vi "Map 1st Generation.vi"(8 "error in":errorcluster, 11 "XML Document in":refnum<class "XML Document.lvclass">) -> (0 "error out":errorcluster, 3 "XML Document out":refnum<class "XML Document.lvclass">)   [LabVIEW 2014, in "XML Document.lvclass"]
uses:
  XML Document.lvclass
  Node_class/Node.lvclass
  <vilib>/xml/Close Reference(Node).vi
  <resource>/objmgr/DOMUserDefRef.rc
  Element_class/Element.lvclass
  <vilib>/xml/NI_XML.lvlib
  Text Node_class/Text Node.lvclass
  Comment Node_class/Comment Node.lvclass
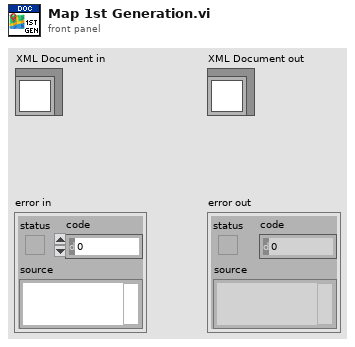
[diagram p1: front panel]
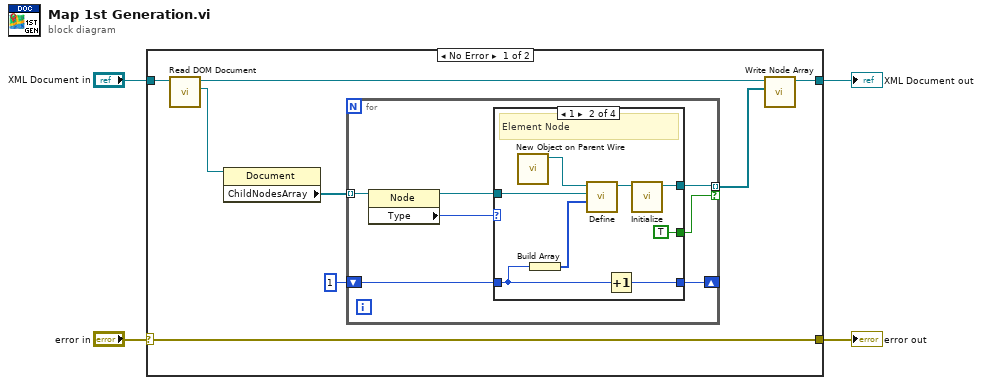
[diagram p0: block diagram]
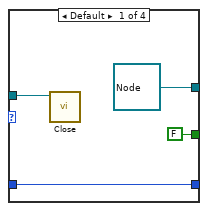
[diagram p2: hidden frame]
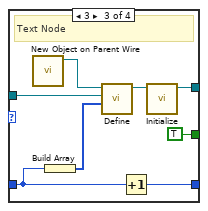
[diagram p3: hidden frame]
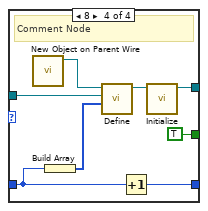
[diagram p4: hidden frame]
diagram:
  n1 = case shown="No Error" "error in" {
    selector: "error in" -> [w11 w49]
    tunnel: [w11 w49] -> w3
    tunnel: [w6 w48] -> w1
    tunnel: "XML Document in" -> [w12 w48]
    frame No Error {
      n2 = call-dynamic "Read DOM Document.vi"("XML Document in"=w12) -> ("DOM Document"=w9:refnum<k20>, "XML Document out"=w10:refnum<class "XML Document.lvclass">)  [unwired: 8 in, 1 out]
      n3 = property class="Document"(reference=w9) -> ("ChildNodesArray"=w8:refnum<k20>[])  [unwired: 1 in, 2 out]
      n4 = for {
        tunnel: w8 -> [w19] mode=indexing
        shift-right: [w15] -> _
        shift-left: 1 ("Address Location Part") -> [w16]
        tunnel: [w14] -> w5 mode=indexing if=w13
        n5 = property class="Node"(reference=w19) -> (reference out=w18:refnum<k20>, "Type"=w17:i32)  [unwired: 1 in, 1 out]
        n6 = case shown="1" w17 {
          tunnel: w18 -> [w20 w29 w37 w45]
          tunnel: w16 -> [w23 w31 w39 w47]
          tunnel: [w23 w30 w38 w46] -> w15
          tunnel: [refnum<class "Node.lvclass"> refnum ("Node out") w24 w33 w41] -> w14
          tunnel: [FALSE TRUE TRUE TRUE] -> w13
          frame Default {
            n7 = call-poly <vilib>:"Close.vi"("node"=w20) -> ()  [unwired: 8 in, 1 out]
          }
          frame 1 {
            # "Element Node"
            n8 = call "New Object on Parent Wire.vi"() -> ("Node.lvclass"=w27:refnum<class "Node.lvclass">)  [unwired: 10 in, 1 out]
            n9 = Build Array(w31) -> (w28:i32[])
            n10 = call-dynamic "Define.vi"("Address"=w28, "Node Refnum"=w29, "Node in"=w27) -> ("Node out"=w26:refnum<class "Node.lvclass">)  [unwired: 7 in, 1 out]
            n11 = Increment(x=w31) -> (x+1=w30:i32)
            n12 = call-dynamic "Initialize.vi"("Node in"=w26) -> ("Node out"=w24:refnum<class "Node.lvclass">)  [unwired: 9 in, 1 out]
          }
          frame 3 {
            # "Text Node"
            n13 = call "New Object on Parent Wire.vi"() -> ("Node.lvclass"=w35:refnum<class "Node.lvclass">)  [unwired: 10 in, 1 out]
            n14 = Build Array(w39) -> (w36:i32[])
            n15 = call-dynamic "Define.vi"("Address"=w36, "Node Refnum"=w37, "Node in"=w35) -> ("Node out"=w34:refnum<class "Node.lvclass">)  [unwired: 7 in, 1 out]
            n16 = Increment(x=w39) -> (x+1=w38:i32)
            n17 = call-dynamic "Initialize.vi"("Node in"=w34) -> ("Node out"=w33:refnum<class "Node.lvclass">)  [unwired: 9 in, 1 out]
          }
          frame 8 {
            # "Comment Node"
            n18 = call "New Object on Parent Wire.vi"() -> ("Node.lvclass"=w43:refnum<class "Node.lvclass">)  [unwired: 10 in, 1 out]
            n19 = Build Array(w47) -> (w44:i32[])
            n20 = call-dynamic "Define.vi"("Address"=w44, "Node Refnum"=w45, "Node in"=w43) -> ("Node out"=w42:refnum<class "Node.lvclass">)  [unwired: 7 in, 1 out]
            n21 = Increment(x=w47) -> (x+1=w46:i32)
            n22 = call-dynamic "Initialize.vi"("Node in"=w42) -> ("Node out"=w41:refnum<class "Node.lvclass">)  [unwired: 9 in, 1 out]
          }
        }
      }
      n23 = call-dynamic "Write Node Array.vi"("Node Array"=w5, "XML Document in"=w10) -> ("XML Document out"=w6:refnum<class "XML Document.lvclass">)  [unwired: 8 in, 1 out]
    }
    frame Error {
    }
  }
  "error out" <- w3
  "XML Document out" <- w1
